vi "emulate cursor.vi"(0 "Display":refnum<vi>, 1 "This VI":refnum<vi>, 5 "Selection":cluster{i32, i32}, 7 "Highlighted String":string, 9 "Cursor":cluster{i32, i32}, 11 "error in":errorcluster) -> (15 "error out":errorcluster)   [LabVIEW 2018]
uses:
  <vilib>/Utility/miscctls.llb/LVRowAndColumnTypeDef.ctl
panel:
  out "selection":cluster{i32, i32}
  out "cursor":cluster{i32, i32}
  in  "Highlighted lines":i32[](array[numeric])
  in  "Highlighted text":string[](array[string])
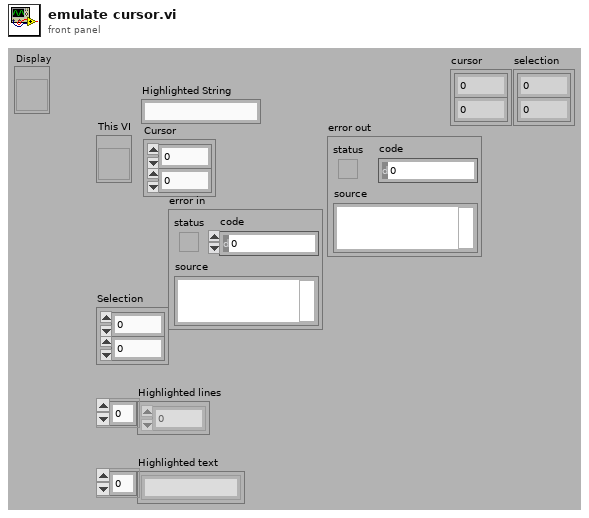
[diagram p1: front panel]
types:
  T1 = typedef "LVRowAndColumnTypeDef.ctl" = cluster{"Row":i32, "Column":i32}
  T2 = typedef "LVRectTypeDef.ctl" = cluster{"Left":i16, "Top":i16, "Right":i16, "Bottom":i16}
  T3 = typedef "LVBoundsTypeDef.ctl" = cluster{"Width":u32, "Height":u32}
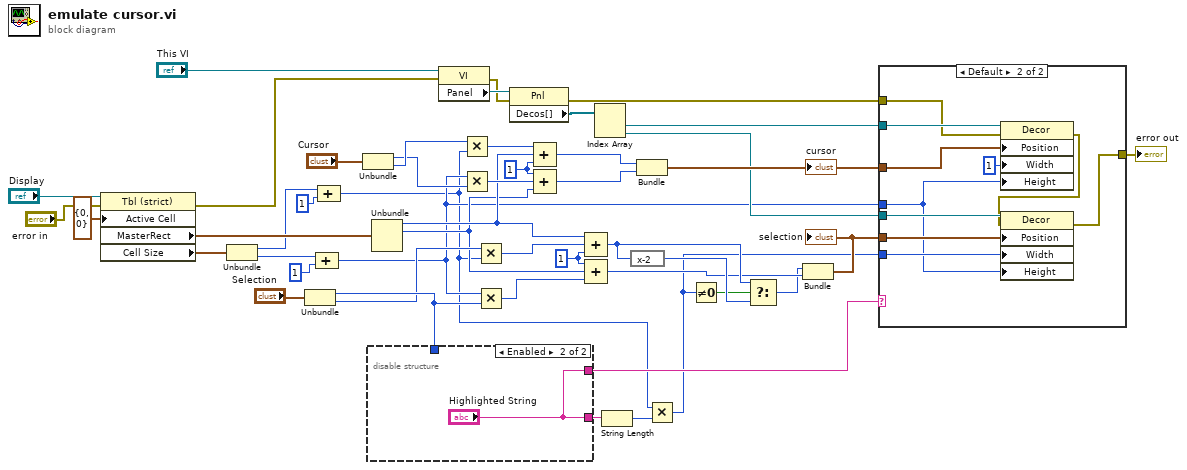
[diagram p0: block diagram]
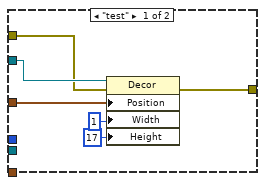
[diagram p2: hidden frame]
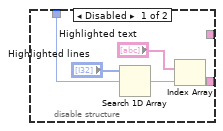
[diagram p3: hidden frame]
diagram:
  w9 = u32 1 ("value")
  w10 = u32 1 ("value")
  n1 = property on="Property Node" class="Tbl (strict)"(reference="Display", error in="error in", "Active Cell"=T1 {"Row"=0, "Column"=0} ("Active Cell:Active Cell")) -> (error out=w21:errorcluster, "MasterRect"=w38:T2, "Cell Size"=w13:T3)  [unwired: 1 out]
  n2 = Unbundle(w13) -> ("Width"=w2:u32, "Height"=w5:u32)
  n3 = Unbundle("Selection") -> (w23:i32, w22:i32)
  n4 = Compound Arithmetic op=ADD(w5, u32 1 ("value")) -> (w4:u32)
  n5 = Compound Arithmetic op=ADD(w2, u32 1 ("value")) -> (w1:u32)
  n6 = Unbundle("Cursor") -> (w24:i32, w25:i32)
  n7 = disable-structure shown="Enabled" {
    disable-tunnel: [w52 "Highlighted String"] -> w44
    disable-tunnel: w23 -> [w49 _]
    disable-tunnel: [_ "Highlighted String"] -> w34
    frame Disabled {
      n8 = Search 1D Array(1D array="Highlighted lines", element=w49) -> (index of element=w50:i32)  [unwired: 1 in]
      n9 = Index Array(array="Highlighted text", index=w50) -> (element=w52:string)
    }
    frame Enabled {
    }
  }
  n10 = Unbundle(w38) -> ("Left"=w8:i16, "Top"=w7:i16)  [unwired: 2 out]
  n11 = property class="VI"(reference="This VI", error in=w21) -> (error out=w20:errorcluster, "Panel"=w36:refnum<vi>)  [unwired: 1 out]
  n12 = Multiply(x=w25, y=w1) -> (x*y=w27:u32)
  n13 = Multiply(x=w4, y=w24) -> (x*y=w26:u32)
  n14 = Multiply(x=w22, y=w1) -> (x*y=w43:u32)
  n15 = Multiply(x=w4, y=w23) -> (x*y=w42:u32)
  n16 = property class="Pnl"(reference=w36, error in=w20) -> (error out=w19:errorcluster, "Decos[]"=w37:refnum<vi>[])  [unwired: 1 out]
  n17 = Compound Arithmetic op=ADD(w27, w8, w9) -> (w29:u32)
  n18 = Compound Arithmetic op=ADD(w9, w26, w7) -> (w28:u32)
  n19 = Compound Arithmetic op=ADD(w8, w43, w10) -> (w46:u32)
  n20 = Compound Arithmetic op=ADD(w10, w7, w42) -> (w41:u32)
  n21 = Index Array(array=w37) -> (element #1=w31:refnum<vi>, element #2=w30:refnum<vi>)  [unwired: 2 in]
  n22 = String Length(string=w44) -> (length=w45:i32)
  n23 = expression code="x-2"(w46) -> (w47:u32)
  n24 = Bundle(w29, w28) -> (w32:cluster{u32, u32})  [unwired: 1 in]
  "cursor" <- w32
  n25 = Multiply(x=w1, y=w45) -> (x*y=w14:u32)
  n26 = Not Equal To 0?(x=w14) -> (x != 0?=w15:bool)
  n27 = Select(t=w46, s=w15, f=w47) -> (s? t:f=w16:u32)
  n28 = Bundle(w16, w41) -> (w40:cluster{u32, u32})  [unwired: 1 in]
  "selection" <- w40
  n29 = case shown="Default" w34 {
    tunnel: w14 -> [_ w69]
    tunnel: w40 -> [_ w68]
    tunnel: w30 -> [_ w67]
    tunnel: w31 -> [w56 w66]
    tunnel: w32 -> [w57 w65]
    tunnel: w19 -> [w55 w63]
    tunnel: [w54 w61] -> w18
    tunnel: w4 -> [_ w60]
    frame "test" {
      n30 = property class="Decor"(reference=w56, error in=w55, "Position"=w57, "Width"=u32 1 ("Size:Width"), "Height"=17 ("x")) -> (error out=w54:errorcluster)  [unwired: 1 out]
    }
    frame Default {
      n31 = property class="Decor"(reference=w66, error in=w63, "Position"=w65, "Width"=u32 1 ("Size:Width"), "Height"=w60) -> (error out=w62:errorcluster)  [unwired: 1 out]
      n32 = property class="Decor"(reference=w67, error in=w62, "Position"=w68, "Width"=w69, "Height"=w60) -> (error out=w61:errorcluster)  [unwired: 1 out]
    }
  }
  "error out" <- w18
